vi "PositionToReceiveRollSkill.vi"(7 "Game in":refnum<class "Game.lvclass">, 8 "error in (no error)":errorcluster, 10 "Robot":refnum<class "Robot.lvclass">, 11 "PositionToReceiveRollSkill in":refnum<class "PositionToReceiveRollSkill.lvclass">) -> (0 "error out":errorcluster, 2 "Robot out":refnum<class "Robot.lvclass">, 3 "PositionToReceiveRollSkill out":refnum<class "PositionToReceiveRollSkill.lvclass">)   [LabVIEW 2021, in "PositionToReceiveRollSkill.lvclass"]
uses:
  PositionToReceiveRollSkill.lvclass
  Game_class/Game.lvclass
  Robot_class/Robot.lvclass
  Game_class/Game.lvclass/Game.ctl
  Object_class/Object.lvclass/Object.ctl
  Parameters_class/Parameters.lvclass/Parameters.ctl
  Robot_class/Robot.lvclass/Robot.ctl
  Game_class/Read FieldRef.vi
  Game_class/Read BallRef.vi
  Game_class/Read Utilities.lvclass.vi
  Game_class/Read Parameters.lvclass.vi
  Parameters_class/Read AttakingOurselves.vi
  Parameters_class/Read DistanceStop.vi
  Object_class/Read x.vi
  Object_class/Read y.vi
  Robot_class/Write dest_x.vi
  Robot_class/Write dest_y.vi
  Robot_class/Write dest_orientation.vi
  Ball_class/Ball.lvclass
  D:/RoboIme/horie/SSL_AI/Object_class/Object.lvclass
  Field_class/Field.lvclass
  Utilities_class/Utilities.lvclass
  Parameters_class/Parameters.lvclass
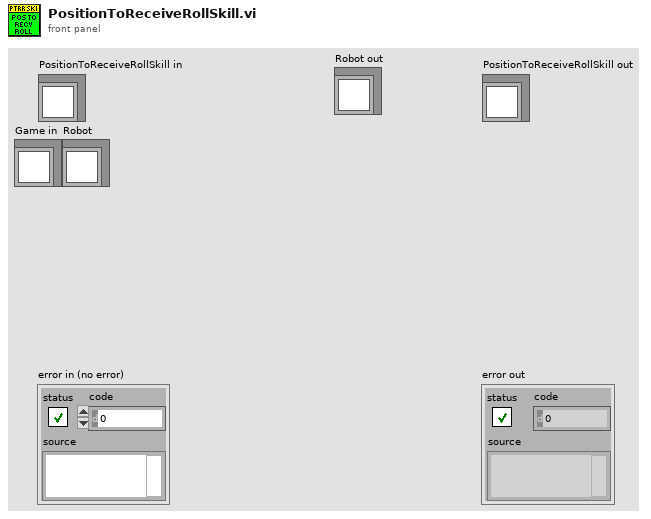
[diagram p1: front panel]
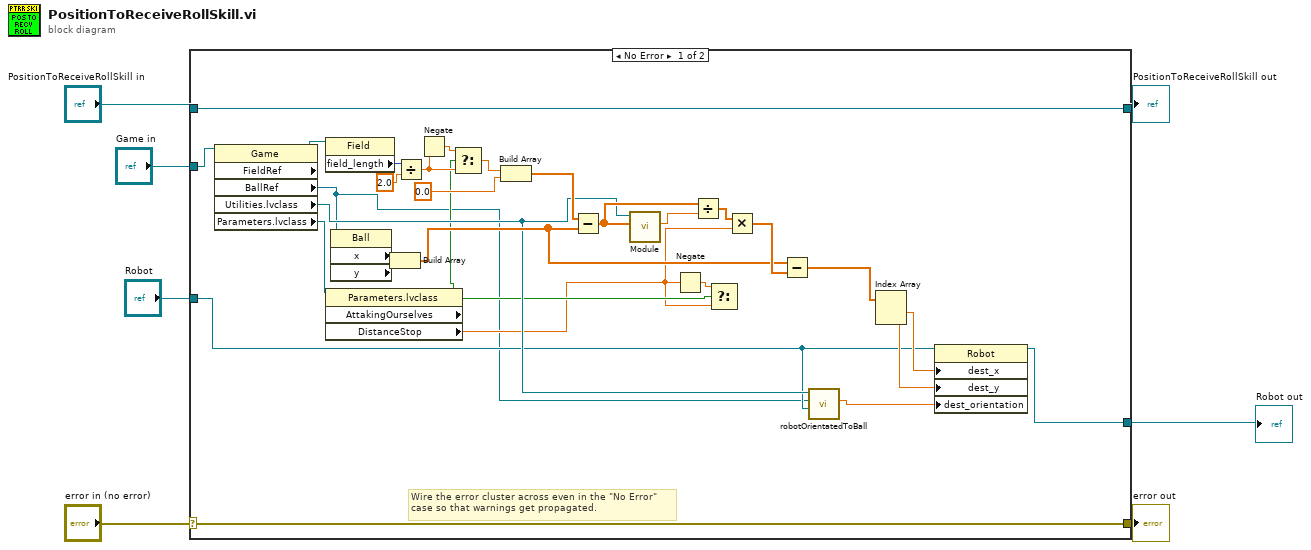
[diagram p0: block diagram]
diagram:
  n1 = case shown="No Error" "error in (no error)" {
    selector: "error in (no error)" -> [w36 w40]
    tunnel: [w36 w40] -> w6
    tunnel: [w37 w39] -> w4
    tunnel: "PositionToReceiveRollSkill in" -> [w37 w39]
    tunnel: "Game in" -> [w8 _]
    tunnel: "Robot" -> [w18 w38]
    tunnel: [w16 w38] -> w1
    frame No Error {
      # "Wire the error cluster across even in the \"No Error\"\ncase so that warnings get propagated."
      n2 = property class="Game"(reference=w8) -> ("FieldRef"=w33:refnum<class "Field.lvclass">, "BallRef"=w9:refnum<class "Ball.lvclass">, "Utilities.lvclass"=w19:refnum<class "Utilities.lvclass">, "Parameters.lvclass"=w26:refnum<class "Parameters.lvclass">)  [unwired: 1 in, 2 out]
      n3 = property class="Field"(reference=w33) -> ("field_length"=w32:i32)  [unwired: 1 in, 2 out]
      n4 = property class="Parameters.lvclass"(reference=w26) -> ("AttakingOurselves"=w12:bool, "DistanceStop"=w10:dbl)  [unwired: 1 in, 2 out]
      n5 = property class="Ball"(reference=w9) -> ("x"=w35:dbl, "y"=w34:dbl)  [unwired: 1 in, 2 out]
      n6 = Build Array(w35, w34) -> (w23:dbl[])
      n7 = Divide(x=w32, y=2.0) -> (x/y=w14:dbl)
      n8 = Negate(x=w14) -> (-x=w15:dbl)
      n9 = Select(t=w15, s=w12, f=w14) -> (s? t:f=w11:dbl)
      n10 = Build Array(w11, 0.0) -> (w29:dbl[])
      n11 = Subtract(x=w29, y=w23) -> (x-y=w28:dbl[])
      n12 = call "Module.vi"("2D vector"=w28, "Utilities in"=w19) -> ("Modulo"=w27:dbl)  [unwired: 7 in, 2 out]
      n13 = Negate(x=w10) -> (-x=w13:dbl)
      n14 = Divide(x=w28, y=w27) -> (x/y=w25:dbl[])
      n15 = Select(t=w13, s=w12, f=w10) -> ()  [unwired: 1 out]
      n16 = Multiply(x=w25, y=w10) -> (x*y=w24:dbl[])
      n17 = Subtract(x=w23, y=w24) -> (x-y=w22:dbl[])
      n18 = call "robotOrientatedToBall.vi"("Robot"=w18, "BallRef"=w9, "Utilities in"=w19) -> ("Orientation"=w17:dbl)  [unwired: 6 in, 2 out]
      n19 = Index Array(array=w22) -> (element #1=w21:dbl, element #2=w20:dbl)  [unwired: 2 in]
      n20 = property class="Robot"(reference=w18, "dest_x"=w21, "dest_y"=w20, "dest_orientation"=w17) -> (reference out=w16:refnum<class "Robot.lvclass">)  [unwired: 1 in, 1 out]
    }
    frame Error {
    }
  }
  "error out" <- w6
  "PositionToReceiveRollSkill out" <- w4
  "Robot out" <- w1
